vi "set_histogram_cursors.vi"(8 "error in (no error)":errorcluster, 9 "Max pos":dbl, 10 "Min pos":dbl, 11 "Histogram reference in":refnum<vi>) -> (0 "error out":errorcluster)   [LabVIEW 2011, in "Fiberscope_library.lvlib"]
uses:
  Fiberscope_library.lvlib
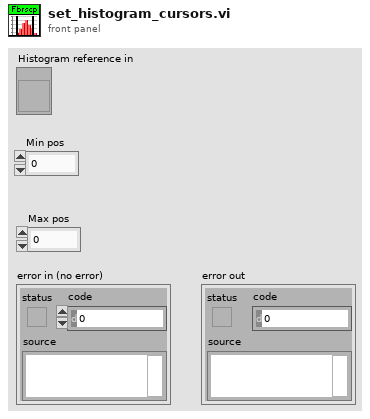
[diagram p1: front panel]
types:
  T1 = typedef "LVCursorListTypeDef.ctl" = cluster{"Name":string, "Color":u32, "Style":u8, "Point Style":u8, "Name Visible":bool, "Allow Drag":bool, "Cursor Mode":u32, "Plot":i32, "Index":i32, "Position":cluster{"X":dbl, "Y":dbl}, "X Scale":u32, "Y Scale":u32, "Watch Plots":i32[], "Watch All Plots":bool, "Plot Area":i32, "Label Offset":cluster{"X":dbl, "Y":dbl}}[]
  T2 = cluster{"Name":string, "Color":u32, "Style":u8, "Point Style":u8, "Name Visible":bool, "Allow Drag":bool, "Cursor Mode":u32, "Plot":i32, "Index":i32, "Position":cluster{"X":dbl, "Y":dbl}, "X Scale":u32, "Y Scale":u32, "Watch Plots":i32[], "Watch All Plots":bool, "Plot Area":i32, "Label Offset":cluster{"X":dbl, "Y":dbl}}
  T3 = cluster{"Name":string, "Color":u32, "Style":u8, "Point Style":u8, "Name Visible":bool, "Allow Drag":bool, "Cursor Mode":u32, "Plot":i32, "Index":i32, "Position":cluster{"X":dbl, "Y":dbl}, "X Scale":u32, "Y Scale":u32, "Watch Plots":i32[], "Watch All Plots":bool, "Plot Area":i32, "Label Offset":cluster{"X":dbl, "Y":dbl}}[]
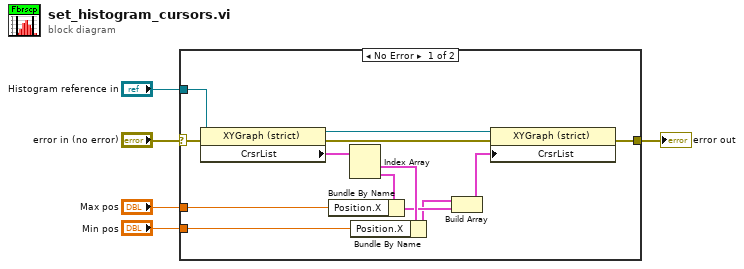
[diagram p0: block diagram]
diagram:
  n1 = case shown="No Error" "error in (no error)" {
    selector: "error in (no error)" -> [w6 w19]
    tunnel: [w17 w19] -> w5
    tunnel: "Min pos" -> [w15 _]
    tunnel: "Max pos" -> [w14 _]
    tunnel: "Histogram reference in" -> [w8 _]
    frame No Error {
      n2 = property on="Property Node" class="XYGraph (strict)"(reference=w8, error in=w6) -> (reference out=w7:refnum<vi>, error out=w16:errorcluster, "CrsrList"=w13:T1)
      n3 = Index Array(array=w13) -> (element #1=w12:T2, element #2=w9:T2)  [unwired: 2 in]
      n4 = Bundle By Name(cluster=w9, "Position.X"=w14) -> (w11:T2)
      n5 = Bundle By Name(cluster=w12, "Position.X"=w15) -> (w10:T2)
      n6 = Build Array(w10, w11) -> (w18:T3)
      n7 = property on="Property Node" class="XYGraph (strict)"(reference=w7, error in=w16, "CrsrList"=w18) -> (error out=w17:errorcluster)  [unwired: 1 out]
    }
    frame Error {
    }
  }
  "error out" <- w5
